vi "Write SequenceConfig.vi"(8 "error in (no error)":errorcluster, 10 "Sequence Config.lvclass":refnum<class "Sequence Config.lvclass">, 11 "SequenceRepo in":refnum<class "SequenceRepo.lvclass">) -> (0 "error out":errorcluster, 3 "SequenceRepo out":refnum<class "SequenceRepo.lvclass">)   [LabVIEW 2015, in "SequenceRepo.lvclass"]
uses:
  SequenceRepo.lvclass
  Prototype/classes/Sequence/Config/Sequence Config.lvclass
  SequenceRepo.lvclass/SequenceRepo.ctl
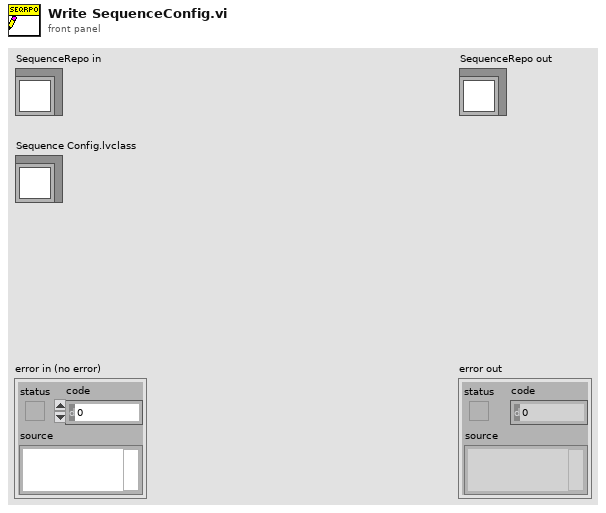
[diagram p1: front panel]
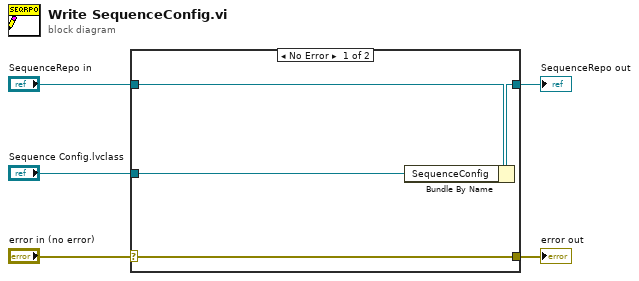
[diagram p0: block diagram]
diagram:
  n1 = case shown="No Error" "error in (no error)" {
    selector: "error in (no error)" -> [w9 w10]
    tunnel: [w9 w10] -> w4
    tunnel: [w7 w11] -> w2
    tunnel: "SequenceRepo in" -> [w8 w11]
    tunnel: "Sequence Config.lvclass" -> [w6 _]
    frame No Error {
      n2 = Bundle By Name(cluster=w8, "SequenceConfig"=w6) -> (w7:refnum<class "SequenceRepo.lvclass">)
    }
    frame Error {
    }
  }
  "error out" <- w4
  "SequenceRepo out" <- w2
